vi "SV TDMS Read Order Level Components (NxM).vi"(0 "tdms file":refnum<k34>, 5 "group name in":string, 7 "channel names in":string[][](array[string]), 11 "error in":errorcluster) -> (3 "scale labels":T1, 4 "tdms file out":refnum<k34>, 6 "group name out":string, 8 "channel names out":string[][](array[string]), 10 "order components":cluster{"X":dbl[], "Y":dbl[]}[][](array[cluster]), 13 "spectra info":T2[](array[typedef]) {"x-axis units" items=["Time (s)"=0, "Frequency-CB (Hz)"=1, "Frequency-CPB (Hz)"=1248, "Frequency-Arbitrary (Hz)"=2357, "Quefrency (s)"=2, "Revolutions (rev)"=3, "Order"=4, "Speed (RPM)"=11, "Speed (rad/s)"=21, "Index"=65535]; "weighting filter" items=["Linear", "A-weighting", "B-weighting", "C-weighting", "ITU-R 468-4", "Dolby", "CCITT", "C-message", "Wb", "Wc", "Wd", "We", "Wf", "Wh", "Wj", "Wk", "Wm", "AES17 20 kHz lowpass", "AES17 40 kHz lowpass", "AES17 20 kHz highpass", "AES17 40 kHz highpass"]; "dB reference [EU]" format="%.2f"; "engineering units" items=["custom..."=0, "V"=1, "A"=21, "C"=30, "pC"=31, "s"=32, "-"=29, "Pa"=2, "N"=20, "g"=3, "m/s^2"=4, "m/s"=5, "m"=6, "mm/s"=12, "mm"=13, "micron/s"=14, "micron"=15, "in/s^2"=7, "in/s"=8, "in"=9, "mil/s"=10, "mil"=11, "rad/s^2"=16, "rad/s"=17, "rad"=18, "deg/s^2"=26, "deg/s"=27, "deg"=28, "RPM"=22, "cycle/s^2"=23, "Hz"=24, "cycle"=25, "strain"=19]; "spectral info"."window" items=["None "=0, "Hanning"=1, "Hamming"=2, "Blackman-Harris"=3, "Exact Blackman"=4, "Blackman"=5, "Flat Top"=6, "4 Term B-Harris "=7, "7 Term B-Harris"=8, "Low Sidelobe"=9, "Force - Exponential"=10, "Gaussian"=62]}, 15 "error out":errorcluster)   [LabVIEW 2017]
doc: "Reads the specified .tdms file and returns data in a format specific to the polymorphic instance selected."
uses:
  <vilib>/addons/_NISVFA/_Shared subVIs/Controls/svc_Spectrum Info.ctl
  <vilib>/addons/_NISVFA/_Shared subVIs/Controls/svc_X-Axis Units.ctl
  <vilib>/addons/_NISVFA/_Shared subVIs/Controls/svc_Spectrum Type.ctl
  <vilib>/addons/_NISVFA/_Shared subVIs/Controls/svc_Engineering Units Text Ring.ctl
  <vilib>/addons/_NISVFA/_Shared subVIs/Controls/svc_Weighting Filter Text Ring.ctl
  <vilib>/addons/_NISVFA/_Shared subVIs/Controls/svc_Complimentary Spectrum Units.ctl
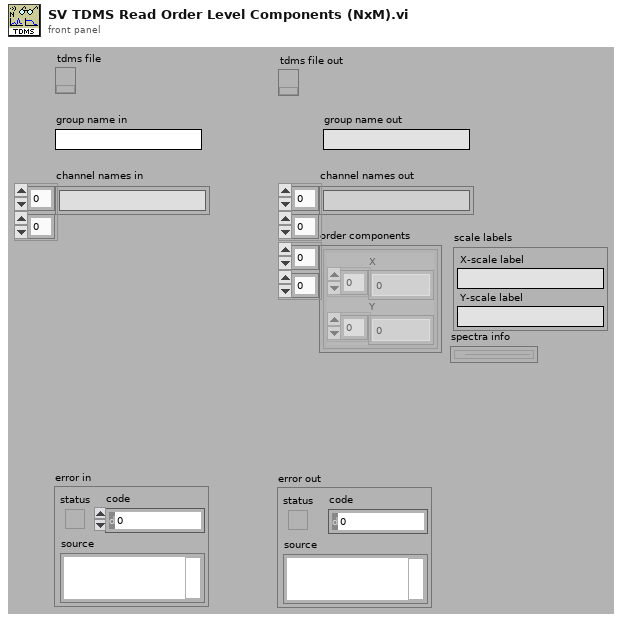
[diagram p1: front panel]
types:
  T1 = cluster{"X-scale label":string, "Y-scale label":string}
  T2 = typedef "svc_Spectrum Info.ctl" = cluster{"channel name":string, "description":string, "x-axis units":T3, "spectral info":cluster{"spectrum type":T4, "linear/dB":enum16{"linear", "dB"}, "window":u16, "window size":i32, "FFT size":i32}, "engineering units":T5, "custom label":string, "dB reference [EU]":dbl, "peak units":enum16{"rms", "peak", "peak-peak"}, "weighting filter":T6, "spectral density?":bool, "unit label":string, "spectrum skewed?":bool, "complimentary spectrum units":T7}
  T3 = typedef "svc_X-Axis Units.ctl" = u16
  T4 = typedef "svc_Spectrum Type.ctl" = enum16{"FFT Spectrum [complex]", "Amplitude [Magnitude]", "Power [Magnitude^2]", "Cross Spectrum [complex]", "Frequency Response [Complex]"}
  T5 = typedef "svc_Engineering Units Text Ring.ctl" = u16
  T6 = typedef "svc_Weighting Filter Text Ring.ctl" = u16
  T7 = typedef "svc_Complimentary Spectrum Units.ctl" = enum16{"none", "radians", "degrees", "cycles", "imaginary"}
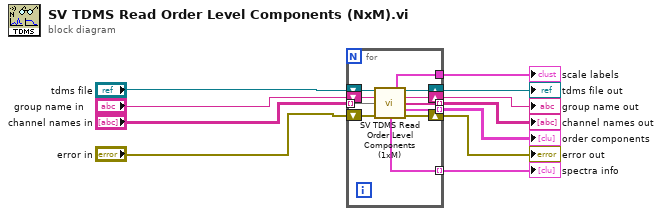
[diagram p0: block diagram]
diagram:
  n1 = for {
    tunnel: "channel names in" -> [w19] mode=indexing
    shift-right: [w22] -> w9
    shift-left: "tdms file" -> [w21]
    shift-right: [w18] -> w2
    shift-left: "group name in" -> [w20]
    tunnel: [w17] -> w3 mode=indexing
    shift-right: [w15] -> w5
    shift-left: "error in" -> [w16]
    tunnel: [w14] -> w4 mode=indexing
    tunnel: [w12] -> w6 mode=indexing
    tunnel: [w13] -> w1
    n2 = call <vilib>:"SV TDMS Read Order Level Components (1xM).vi"("tdms file"=w21, "group name in"=w20, "channel names in"=w19, "error in"=w16) -> ("scale labels"=w13:T1, "tdms file out"=w22:refnum<k34>, "group name out"=w18:string, "channel names out"=w17:string[], "order components"=w14:cluster{"X":dbl[], "Y":dbl[]}[], "spectrum info"=w12:T2, "error out"=w15:errorcluster)  [unwired: 5 in]
  }
  "error out" <- w5
  "tdms file out" <- w9
  "order components" <- w4
  "group name out" <- w2
  "spectra info" <- w6
  "channel names out" <- w3
  "scale labels" <- w1
